vi "Shunt current (SubVI).vi"(6 "R_sh":dbl, 9 "R_s":dbl, 10 "I":dbl, 11 "V":dbl) -> (3 "I_sh":dbl)   [LabVIEW 2024]
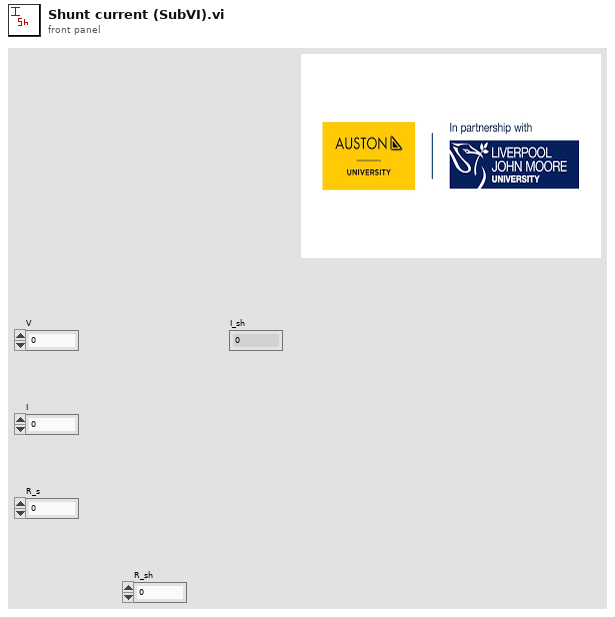
[diagram p1: front panel]
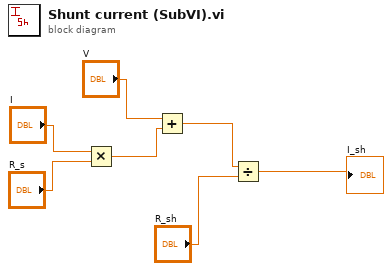
[diagram p0: block diagram]
diagram:
  n1 = Multiply(x="I", y="R_s") -> (x*y=w4:dbl)
  n2 = Add(x="V", y=w4) -> (x+y=w5:dbl)
  n3 = Divide(x=w5, y="R_sh") -> (x/y=→"I_sh":dbl)
